vi "Target Load Cell Read TB 4330.vi"(11 "task/channels in":refnum<k21>) -> (0 "Cable Force (N)":dbl)   [LabVIEW 2018, in "COBRA Measurement and Filtering Library.lvlib"]
uses:
  COBRA Measurement and Filtering Library.lvlib
  <vilib>/DAQmx/read.llb/DAQmx Read (Analog DBL 1Chan 1Samp).vi
  <vilib>/DAQmx/configure/timing.llb/DAQmx Timing (Sample Clock).vi
  <vilib>/DAQmx/miscellaneous.llb/DAQmx Fill In Error Info.vi
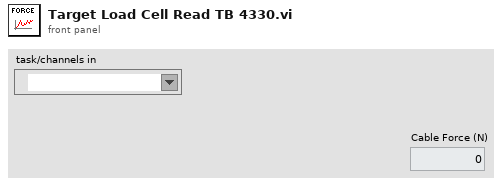
[diagram p1: front panel]
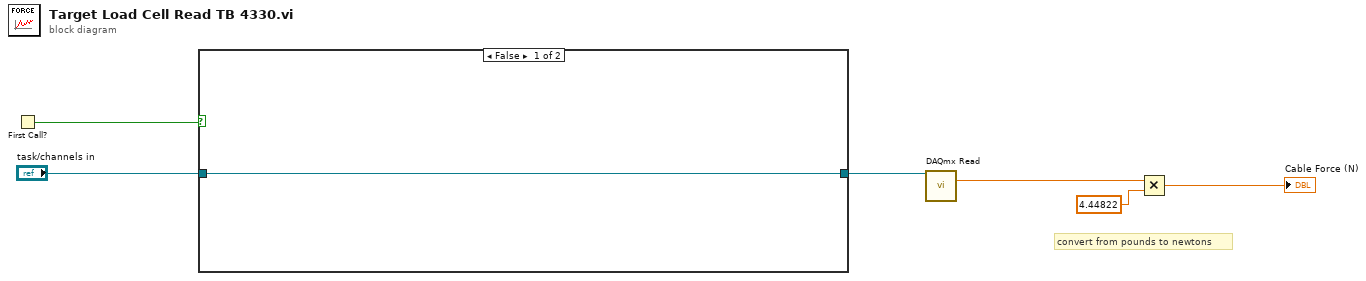
[diagram p0: block diagram]
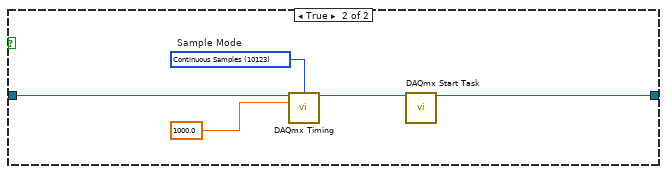
[diagram p2: hidden frame]
diagram:
  # "convert from pounds to newtons"
  n1 = First Call?() -> (First Call?: T/F=w1:bool)
  n2 = case shown="False" w1 {
    tunnel: "task/channels in" -> [w7 w10]
    tunnel: [w7 w12] -> w5
    frame False {
    }
    frame True {
      w11 = 10123 items=["Finite Samples"=10178, "Continuous Samples"=10123, "Hardware Timed Single Point"=12522]  # Sample Mode
      n3 = call-poly <vilib>:"DAQmx Timing.vi"("task/channels in"=w10, "sample mode"=w11, "rate"=1000.0) -> ("task out"=w9:refnum<k21>)  [unwired: 11 in, 1 out]
      n4 = call <vilib>:"DAQmx Start Task.vi"("task/channels in"=w9) -> ("task out"=w12:refnum<k21>)  [unwired: 13 in, 1 out]
    }
  }
  n5 = call-poly <vilib>:"DAQmx Read.vi"("task/channels in"=w5) -> ("data"=w4:dbl)  [unwired: 12 in, 2 out]
  n6 = Multiply(x=w4, y=4.44822 ("Cable Force (N)")) -> (x*y=→"Cable Force (N)":dbl)
